vi "Funnel Finish.vi"   [LabVIEW 2016]
types:
  T1 = typedef "WPI_SolenoidDevRef.ctl" = cluster{"DevStatus":errorcluster, "Pneumatics Control Module":u8, "Forward Solenoid Channel":T2, "Reverse Solenoid Channel":T2}
  T2 = typedef "WPI_SolenoidChannel.ctl" = enum8{"Solenoid 0", "Solenoid 1", "Solenoid 2", "Solenoid 3", "Solenoid 4", "Solenoid 5", "Solenoid 6", "Solenoid 7", "Invalid"}
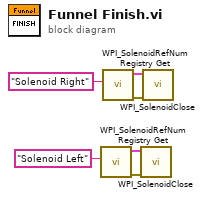
[diagram p0: block diagram]
diagram:
  n1 = call <vilib>:"WPI_SolenoidRefNum Registry Get.vi"("refnum name"="Solenoid Left") -> ("error out"=w4:errorcluster, "SolenoidDevRef"=w3:T1)  [unwired: 9 in]
  n2 = call <vilib>:"WPI_SolenoidRefNum Registry Get.vi"("refnum name"="Solenoid Right") -> ("error out"=w6:errorcluster, "SolenoidDevRef"=w5:T1)  [unwired: 9 in]
  n3 = call <vilib>:"WPI_SolenoidClose.vi"("error in (no error)"=w4, "SolenoidDevRef"=w3) -> ()  [unwired: 9 in, 1 out]
  n4 = call <vilib>:"WPI_SolenoidClose.vi"("error in (no error)"=w6, "SolenoidDevRef"=w5) -> ()  [unwired: 9 in, 1 out]
